vi "Register User Event.vi"(8 "error in (no error)":errorcluster, 10 "Event Registration in":refnum<event-registration>, 11 "Session in":refnum<k21>) -> (0 "error out":errorcluster, 2 "Event Registration out":refnum<event-registration>, 3 "Session out":refnum<k21>)   [LabVIEW 2017, in "nisyscfg.lvlib"]
uses:
  <vilib>/nisyscfg/nisyscfg.lvlib
  <vilib>/nisyscfg/User Event.ctl
panel:
  out "System Configuration":refnum<user-event>
  in  "Target Event":T1
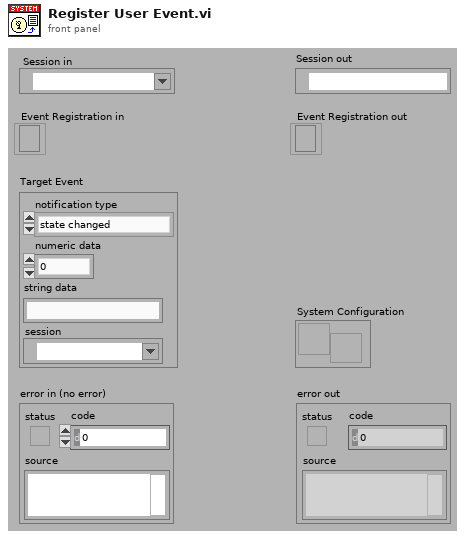
[diagram p1: front panel]
types:
  T1 = typedef "nisyscfg.lvlib/User Event.ctl" = cluster{"notification type":enum32{"state changed", "beginning restart", "getting file", "putting file", "creating directory", "deleting file", "deleting directory", "enumerating file system", "renaming file", "current component", "operation progress", "downloading file", "unpacking file", "running install script", "creating image", "validating image", "applying image", "beginning format", "completing format"}, "numeric data":u32, "string data":string, "session":refnum<k21>}
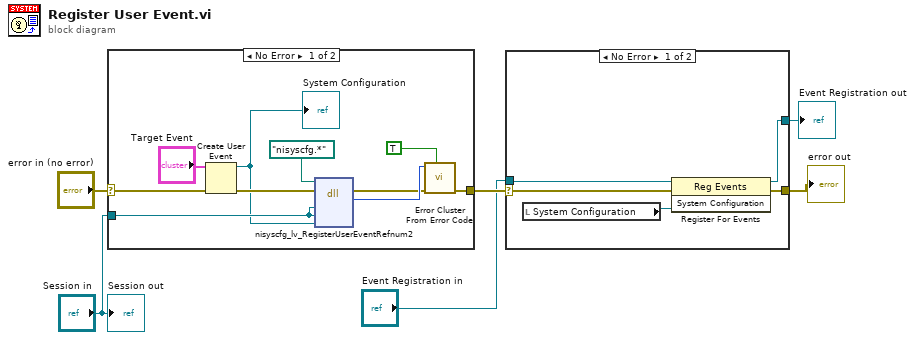
[diagram p0: block diagram]
diagram:
  n1 = case shown="No Error" "error in (no error)" {
    selector: "error in (no error)" -> [w12 w17]
    tunnel: [w8 w17] -> w4
    tunnel: "Session in" -> [w9 _]
    frame No Error {
      n2 = Create User Event(user event datatype="Target Event", error in=w12) -> (user event=w7:refnum<user-event>, error out=w10:errorcluster)
      "System Configuration" <- w7
      n3 = dll-call lib="nisyscfg.*" fn="nisyscfg_lv_RegisterUserEventRefnum2" label="Register User Event"(path in=path "nisyscfg.*", error in=w10, "system"=w9, "session handle"=w9, "event"=w7) -> (error out=w15:errorcluster, "result"=w16:i32)  [unwired: 4 in, 1 out]
      n4 = call <vilib>:"Error Cluster From Error Code.vi"("show call chain? (False)"=TRUE, "error in (no error)"=w15, "error code (0)"=w16) -> ("error out"=w8:errorcluster)  [unwired: 6 in]
    }
    frame Error {
    }
  }
  n5 = case shown="No Error" w4 {
    selector: w4 -> [w22 w24]
    tunnel: [w21 w24] -> w3
    tunnel: [w19 w23] -> w2
    tunnel: "Event Registration in" -> [w18 w23]
    frame No Error {
      n6 = local read "System Configuration"() -> (w20:refnum<user-event>)
      n7 = register-events(reference=w18, error in=w22, w20) -> (reference out=w19:refnum<event-registration>, error out=w21:errorcluster)
    }
    frame Error {
    }
  }
  "error out" <- w3
  "Event Registration out" <- w2
  "Session out" <- "Session in"
